vi "Configure QuickDrop UI.vi"(7 "FP UI References":T1, 8 "error in (no error)":errorcluster, 11 "Test in":refnum<class "Test.lvclass">) -> (0 "error out":errorcluster)   [LabVIEW 2018]
doc: "Dynamically shows or hides the relevant controls on the front panel of the Quick Drop UI, and renames some of the captions for controls to make it perform correctly."
uses:
  FP UI References.ctl
  Test Classes/Test.lvclass
  Comparison Ctrl Refs.ctl
  Comparison Visibility.ctl
  Test Classes/Test Class String IDs.vi
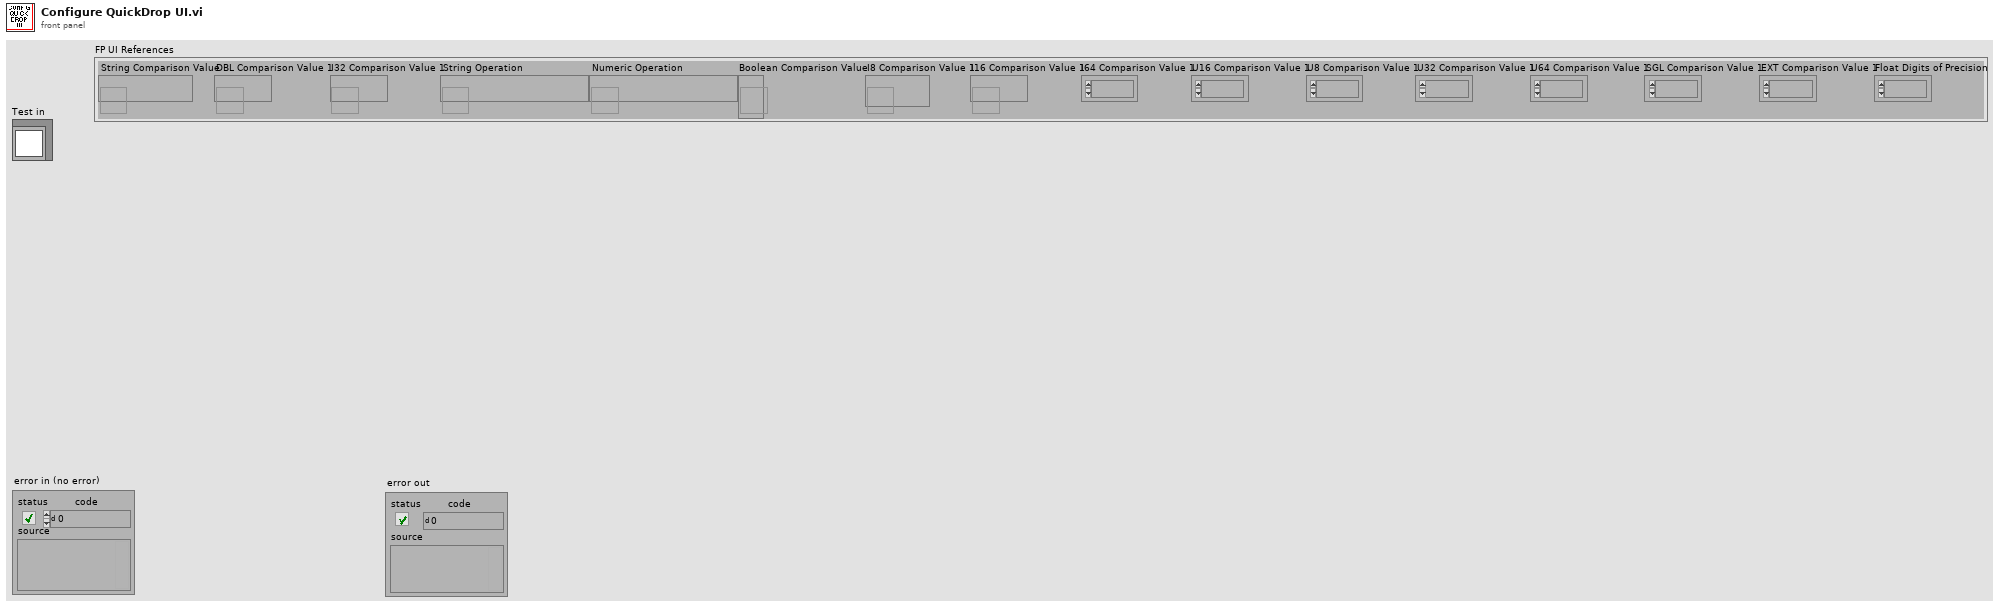
[diagram p1: front panel]
types:
  T1 = typedef "FP UI References.ctl" = cluster{"String Comparison Value":refnum<vi>, "DBL Comparison Value 1":refnum<vi>, "I32 Comparison Value 1":refnum<vi>, "String Operation":refnum<vi>, "Numeric Operation":refnum<vi>, "Boolean Comparison Value":refnum<vi>, "I8 Comparison Value 1":refnum<vi>, "I16 Comparison Value 1":refnum<vi>, "I64 Comparison Value 1":refnum<vi>, "U16 Comparison Value 1":refnum<vi>, "U8 Comparison Value 1":refnum<vi>, "U32 Comparison Value 1":refnum<vi>, "U64 Comparison Value 1":refnum<vi>, "SGL Comparison Value 1":refnum<vi>, "EXT Comparison Value 1":refnum<vi>, "Float Digits of Precision":refnum<vi>}
  T2 = typedef "Comparison Visibility.ctl" = cluster{"Comparison 1 Visible":bool}
  T3 = typedef "Comparison Ctrl Refs.ctl" = cluster{"Comparison Value 1 Control":refnum<vi>}
  T4 = cluster{"Comparison Value 1":string, "Comparison Value 2":string, "Invert Result":string, "Assert VI Name":string, "Data Type":string, "Builder User Name":string, "Build Timestamp":string, "Failure Action":string, "Comment":string, "Assert Name":string, "Description":string, "Evaluation String":string}
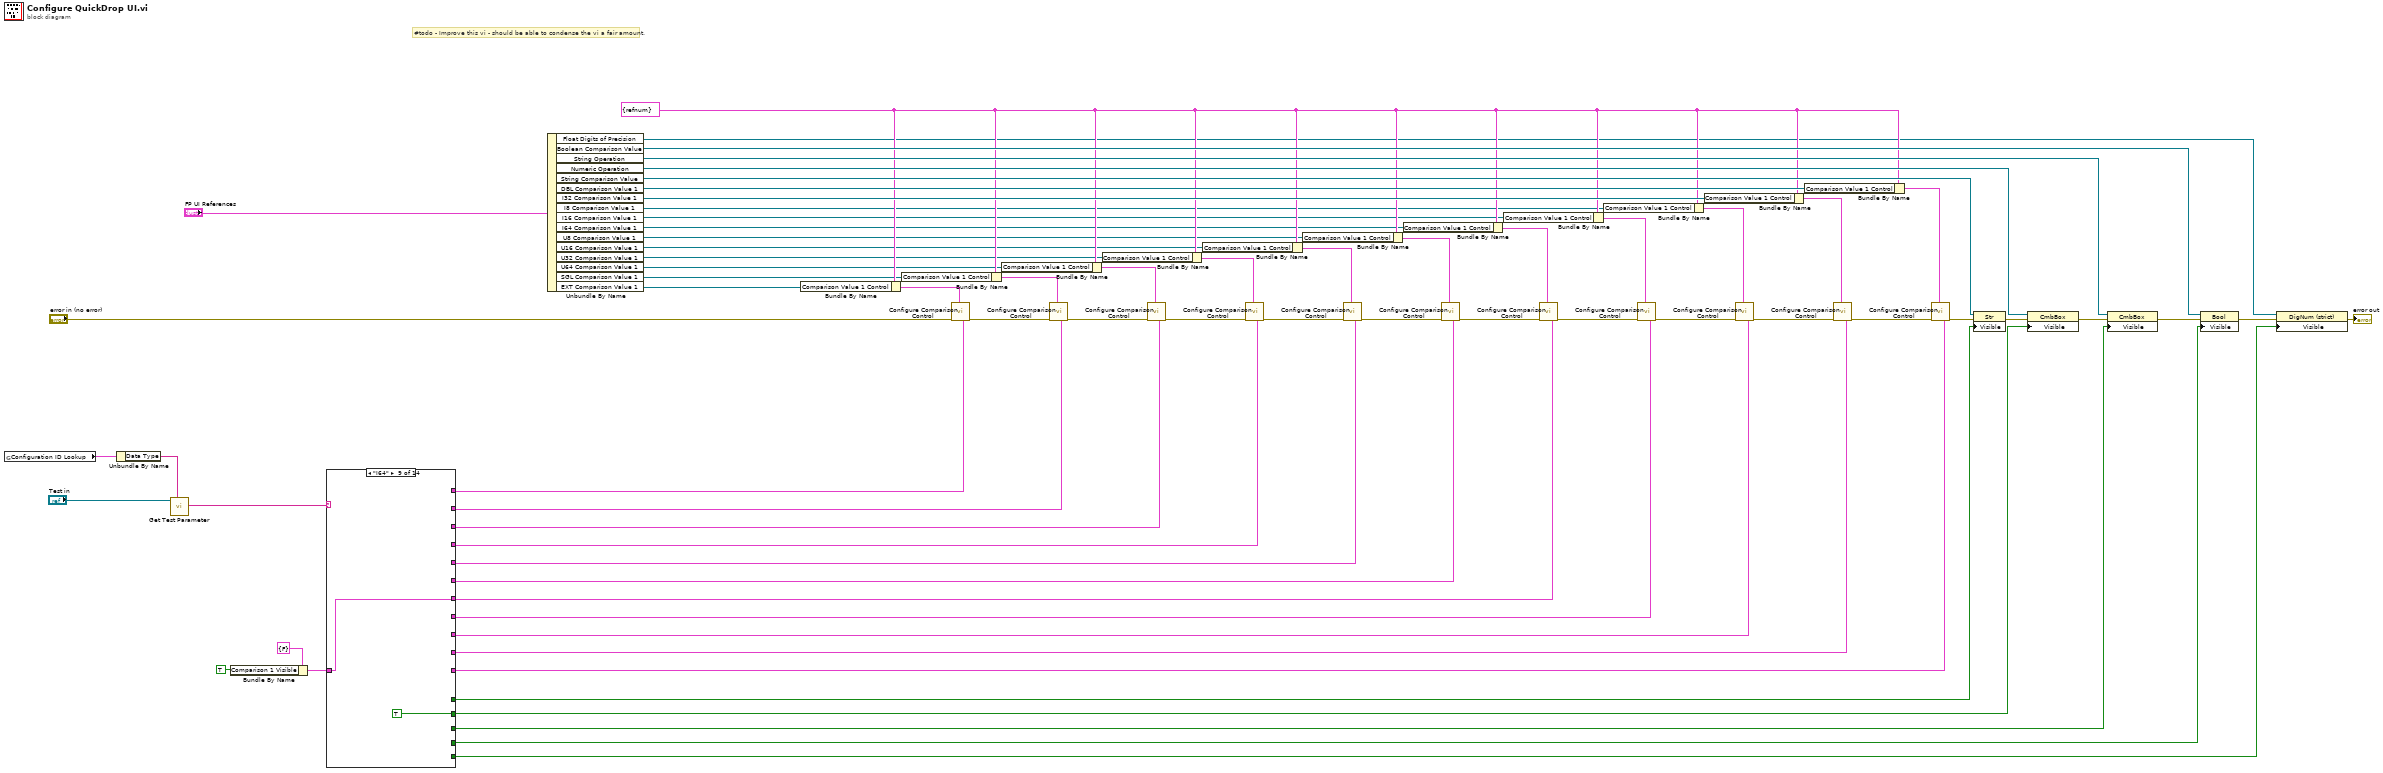
[diagram p0: block diagram]
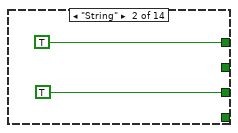
[diagram p3: hidden frame]
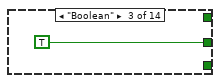
[diagram p4: hidden frame]
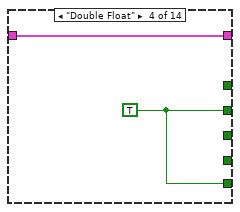
[diagram p5: hidden frame]
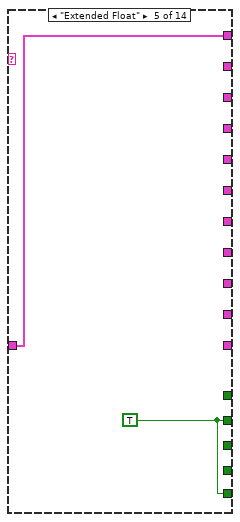
[diagram p6: hidden frame]
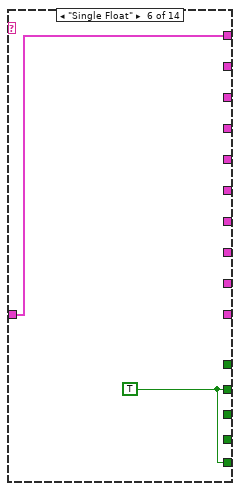
[diagram p7: hidden frame]
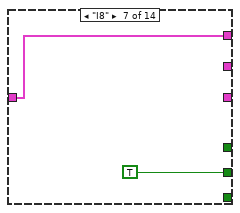
[diagram p8: hidden frame]
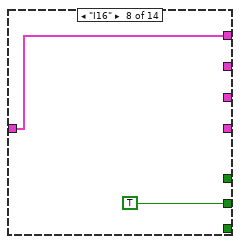
[diagram p9: hidden frame]
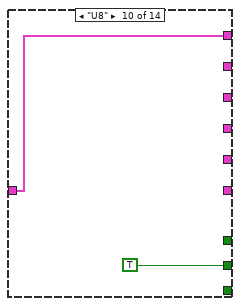
[diagram p10: hidden frame]
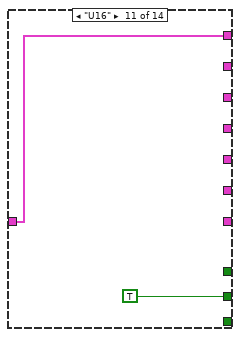
[diagram p11: hidden frame]
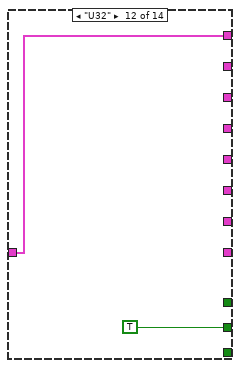
[diagram p12: hidden frame]
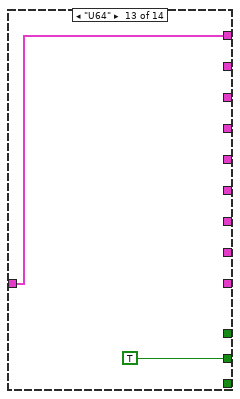
[diagram p13: hidden frame]
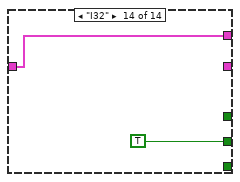
[diagram p14: hidden frame]
diagram:
  w51 = T3 {"Comparison Value 1 Control"=refnum} ("Control Refs")
  # "#todo - Improve this vi - should be able to condense the vi a fair amount."
  n1 = global read "Test Class String IDs.vi" "Configuration ID Lookup"() -> (w4:T4)
  n2 = Unbundle By Name(w4) -> ("Data Type"=w2:string)
  n3 = call "Get Test Parameter.vi"("Data Value ID"=w2, "Test in"="Test in") -> ("Test Parameter"=w1:string)  [unwired: 7 in, 2 out]
  n4 = Bundle By Name(cluster=T2 {"Comparison 1 Visible"=FALSE} ("Control Visibility"), "Comparison 1 Visible"=TRUE) -> (w8:T2)
  n5 = case shown="\"I64\"" w1 {
    tunnel: [_ TRUE _ _ _ _ _ _ _ _ _ _ _ _] -> w64
    tunnel: [_ TRUE _ _ _ _ _ _ _ _ _ _ _ _] -> w60
    tunnel: [_ _ _ w73 w75 w77 TRUE TRUE TRUE TRUE TRUE TRUE TRUE TRUE] -> w59
    tunnel: [_ _ TRUE _ _ _ _ _ _ _ _ _ _ _] -> w55
    tunnel: [_ _ _ _ w76 _ _ _ _ _ _ _ _ _] -> w21
    tunnel: [_ _ _ _ _ w78 _ _ _ _ _ _ _ _] -> w20
    tunnel: [_ _ _ _ _ _ _ _ _ _ _ _ w91 _] -> w19
    tunnel: [_ _ _ _ _ _ _ _ _ _ _ w89 _ _] -> w18
    tunnel: [_ _ _ _ _ _ _ _ _ _ w87 _ _ _] -> w17
    tunnel: [_ _ _ _ _ _ _ _ _ w85 _ _ _ _] -> w16
    tunnel: [_ _ _ _ _ _ _ _ w83 _ _ _ _ _] -> w15
    tunnel: [_ _ _ _ _ _ _ w81 _ _ _ _ _ _] -> w14
    tunnel: [_ _ _ _ _ _ w79 _ _ _ _ _ _ _] -> w13
    tunnel: [_ _ _ _ _ _ _ _ _ _ _ _ _ w93] -> w12
    tunnel: [_ _ _ w74 _ _ _ _ _ _ _ _ _ _] -> w11
    tunnel: w8 -> [_ _ _ w74 w76 w78 w79 w81 w83 w85 w87 w89 w91 w93]
    tunnel: [_ _ _ w73 w75 w77 _ _ _ _ _ _ _ _] -> w5
    frame "Invalid Type", Default {
    }
    frame "String" {
    }
    frame "Boolean" {
    }
    frame "Double Float" {
      w73 = TRUE
    }
    frame "Extended Float" {
      w75 = TRUE
    }
    frame "Single Float" {
      w77 = TRUE
    }
    frame "I8" {
    }
    frame "I16" {
    }
    frame "I64" {
    }
    frame "U8" {
    }
    frame "U16" {
    }
    frame "U32" {
    }
    frame "U64" {
    }
    frame "I32" {
    }
  }
  n6 = Unbundle By Name("FP UI References") -> ("Float Digits of Precision"=w6:refnum<vi>, "Boolean Comparison Value"=w56:refnum<vi>, "String Operation"=w61:refnum<vi>, "Numeric Operation"=w58:refnum<vi>, "String Comparison Value"=w68:refnum<vi>, "DBL Comparison Value 1"=w52:refnum<vi>, "I32 Comparison Value 1"=w54:refnum<vi>, "I8 Comparison Value 1"=w50:refnum<vi>, "I16 Comparison Value 1"=w49:refnum<vi>, "I64 Comparison Value 1"=w48:refnum<vi>, "U8 Comparison Value 1"=w47:refnum<vi>, "U16 Comparison Value 1"=w46:refnum<vi>, "U32 Comparison Value 1"=w45:refnum<vi>, "U64 Comparison Value 1"=w44:refnum<vi>, "SGL Comparison Value 1"=w43:refnum<vi>, "EXT Comparison Value 1"=w42:refnum<vi>)
  n7 = Bundle By Name(cluster=w51, "Comparison Value 1 Control"=w42) -> (w22:T3)
  n8 = Bundle By Name(cluster=w51, "Comparison Value 1 Control"=w43) -> (w24:T3)
  n9 = call "Configure Comparison Control.vi"("Control Visibility"=w21, "Control Refs"=w22, "error in (no error)"="error in (no error)") -> ("error out"=w23:errorcluster)  [unwired: 8 in]
  n10 = Bundle By Name(cluster=w51, "Comparison Value 1 Control"=w44) -> (w25:T3)
  n11 = call "Configure Comparison Control.vi"("Control Visibility"=w20, "Control Refs"=w24, "error in (no error)"=w23) -> ("error out"=w40:errorcluster)  [unwired: 8 in]
  n12 = Bundle By Name(cluster=w51, "Comparison Value 1 Control"=w45) -> (w26:T3)
  n13 = call "Configure Comparison Control.vi"("Control Visibility"=w19, "Control Refs"=w25, "error in (no error)"=w40) -> ("error out"=w33:errorcluster)  [unwired: 8 in]
  n14 = Bundle By Name(cluster=w51, "Comparison Value 1 Control"=w46) -> (w27:T3)
  n15 = call "Configure Comparison Control.vi"("Control Visibility"=w18, "Control Refs"=w26, "error in (no error)"=w33) -> ("error out"=w35:errorcluster)  [unwired: 8 in]
  n16 = Bundle By Name(cluster=w51, "Comparison Value 1 Control"=w47) -> (w28:T3)
  n17 = call "Configure Comparison Control.vi"("Control Visibility"=w17, "Control Refs"=w27, "error in (no error)"=w35) -> ("error out"=w34:errorcluster)  [unwired: 8 in]
  n18 = Bundle By Name(cluster=w51, "Comparison Value 1 Control"=w48) -> (w29:T3)
  n19 = call "Configure Comparison Control.vi"("Control Visibility"=w16, "Control Refs"=w28, "error in (no error)"=w34) -> ("error out"=w39:errorcluster)  [unwired: 8 in]
  n20 = Bundle By Name(cluster=w51, "Comparison Value 1 Control"=w49) -> (w30:T3)
  n21 = call "Configure Comparison Control.vi"("Control Visibility"=w15, "Control Refs"=w29, "error in (no error)"=w39) -> ("error out"=w36:errorcluster)  [unwired: 8 in]
  n22 = Bundle By Name(cluster=w51, "Comparison Value 1 Control"=w50) -> (w31:T3)
  n23 = call "Configure Comparison Control.vi"("Control Visibility"=w14, "Control Refs"=w30, "error in (no error)"=w36) -> ("error out"=w38:errorcluster)  [unwired: 8 in]
  n24 = Bundle By Name(cluster=w51, "Comparison Value 1 Control"=w54) -> (w53:T3)
  n25 = call "Configure Comparison Control.vi"("Control Visibility"=w13, "Control Refs"=w31, "error in (no error)"=w38) -> ("error out"=w37:errorcluster)  [unwired: 8 in]
  n26 = Bundle By Name(cluster=w51, "Comparison Value 1 Control"=w52) -> (w32:T3)
  n27 = call "Configure Comparison Control.vi"("Control Visibility"=w12, "Control Refs"=w53, "error in (no error)"=w37) -> ("error out"=w66:errorcluster)  [unwired: 8 in]
  n28 = call "Configure Comparison Control.vi"("Control Visibility"=w11, "Control Refs"=w32, "error in (no error)"=w66) -> ("error out"=w41:errorcluster)  [unwired: 8 in]
  n29 = property class="Str"(reference=w68, error in=w41, "Visible"=w64) -> (error out=w65:errorcluster)  [unwired: 1 out]
  n30 = property class="CmbBox"(reference=w58, error in=w65, "Visible"=w59) -> (error out=w63:errorcluster)  [unwired: 1 out]
  n31 = property class="CmbBox"(reference=w61, error in=w63, "Visible"=w60) -> (error out=w62:errorcluster)  [unwired: 1 out]
  n32 = property class="Bool"(reference=w56, error in=w62, "Visible"=w55) -> (error out=w57:errorcluster)  [unwired: 1 out]
  n33 = property class="DigNum (strict)"(reference=w6, error in=w57, "Visible"=w5) -> (error out=→"error out":errorcluster)  [unwired: 1 out]
